vi "Hide Console.vi"(8 "error in (no error)":errorcluster, 11 "Handler.UserEvent.Console in":refnum<class "Handler.UserEvent.Console.lvclass">) -> (0 "error out":errorcluster, 3 "Handler.UserEvent.Console out":refnum<class "Handler.UserEvent.Console.lvclass">)   [LabVIEW 2017, in "Error Log.lvlib" / "Handler.UserEvent.Console.lvclass"]
uses:
  Handler.UserEvent.Console.lvclass
  Handler.UserEvent.Console.lvclass/Handler.UserEvent.Console.ctl
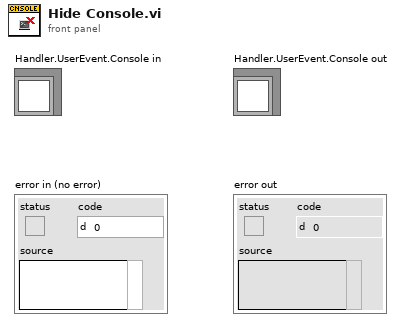
[diagram p1: front panel]
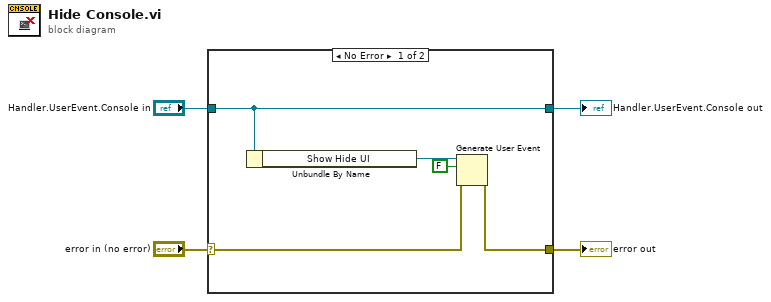
[diagram p0: block diagram]
diagram:
  n1 = case shown="No Error" "error in (no error)" {
    selector: "error in (no error)" -> [w7 w11]
    tunnel: [w6 w11] -> w3
    tunnel: [w9 w10] -> w1
    tunnel: "Handler.UserEvent.Console in" -> [w9 w10]
    frame No Error {
      n2 = Unbundle By Name(w9) -> ("Show Hide UI"=w8:refnum<user-event>)
      n3 = Generate User Event(user event=w8, event data cluster=FALSE ("event data"), error in=w7) -> (error out=w6:errorcluster)  [unwired: 1 in, 1 out]
    }
    frame Error {
    }
  }
  "error out" <- w3
  "Handler.UserEvent.Console out" <- w1
